vi "serial.Write.vi"(7 "serial":T1, 8 "error in":errorcluster, 11 "VISA in":refnum<visa-resource-name>) -> (0 "error out":errorcluster)   [LabVIEW 2020]
uses:
  _controls/serial.ctl
  6b0e8ef9-8a1d-4fce-98aa-063776d6d543.vi
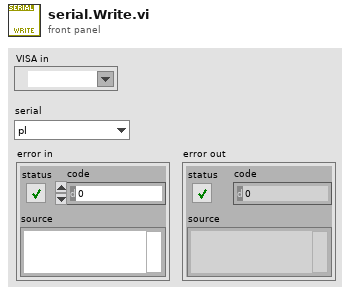
[diagram p1: front panel]
types:
  T1 = typedef "serial.ctl" = enum16{"pl", "idle"}
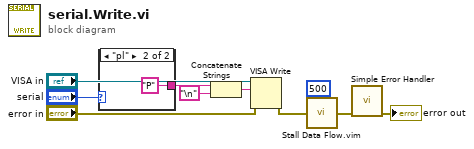
[diagram p0: block diagram]
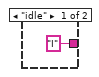
[diagram p2: hidden frame]
diagram:
  n1 = case shown="\"pl\"" "serial" {
    tunnel: ["I" ("string") "P" ("string")] -> w3
    frame "idle" {
    }
    frame "pl" {
    }
  }
  n2 = Concatenate Strings(w3, "\n") -> (w5:string)
  n3 = VISA Write(VISA resource name="VISA in", write buffer=w5, error in (no error)="error in") -> (error out=w7:errorcluster)  [unwired: 2 out]
  n4 = call "Stall Data Flow.vim"("value in"=w7, "milliseconds to wait"=u32 500) -> ("value out"=w2:errorcluster)  [unwired: 1 out]
  n5 = call <vilib>:"Simple Error Handler.vi"("error in (no error)"=w2) -> ("error out"=→"error out":errorcluster)  [unwired: 4 in, 4 out]
